vi "Parse-end-tag-2.vi"(6 "State data in":T1, 8 "error in (no error)":errorcluster, 10 "String in":string, 11 "Element-XML in":refnum<class "Element-XML.lvclass">) -> (0 "error out":errorcluster, 1 "Valid element?":bool, 2 "Remaining string":string, 3 "Element-XML":refnum<class "Element-XML.lvclass">, 4 "State data":T1)   [LabVIEW 2013, in "HardwareCharacterization.lvlib" / "Element-XML.lvclass"]
uses:
  Element-XML.lvclass
  XML-parser-state.ctl
  Element-XML.lvclass/Element-XML.ctl
  Read Parent ItemID.vi
  Read Element.vi
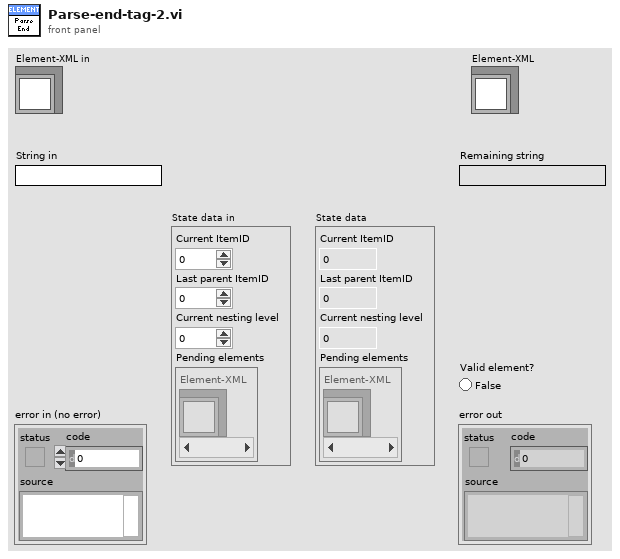
[diagram p1: front panel]
types:
  T1 = typedef "HardwareCharacterization.lvlib/Element-XML.lvclass/XML-parser-state.ctl" = cluster{"Current ItemID":u32, "Last parent ItemID":u32, "Current nesting level":i16, "Pending elements":refnum<class "Element-XML.lvclass">[]}
  T2 = typedef "HardwareCharacterization.lvlib/Element-XML.lvclass/Elements.ctl" = enum16{"BeginJob", "WriteDigital", "WriteAnalog", "Set", "ApplicationEvent", "JumpAbs", "MarkAbs", "JumpRel", "MarkRel", "LongDelay", "EndJob"}
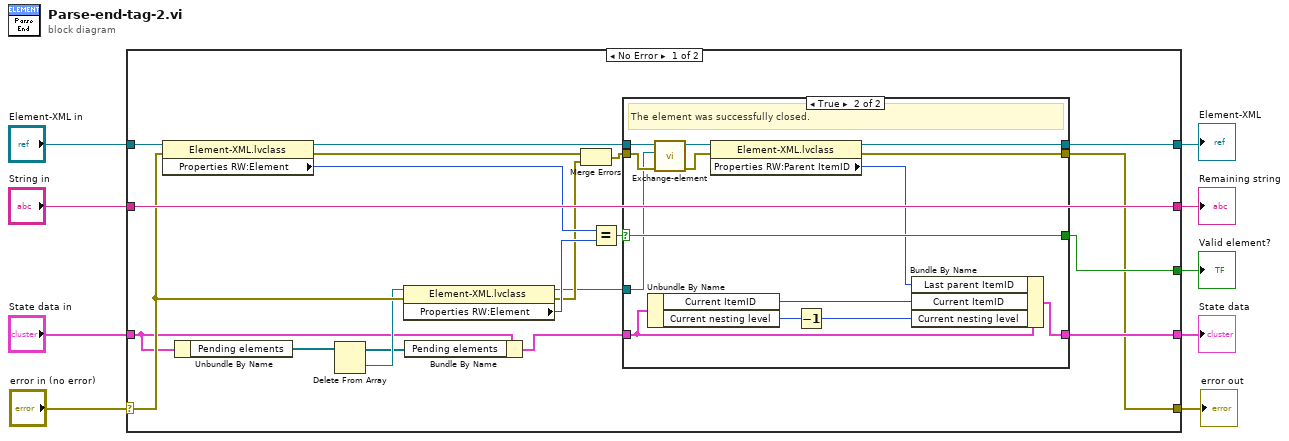
[diagram p0: block diagram]
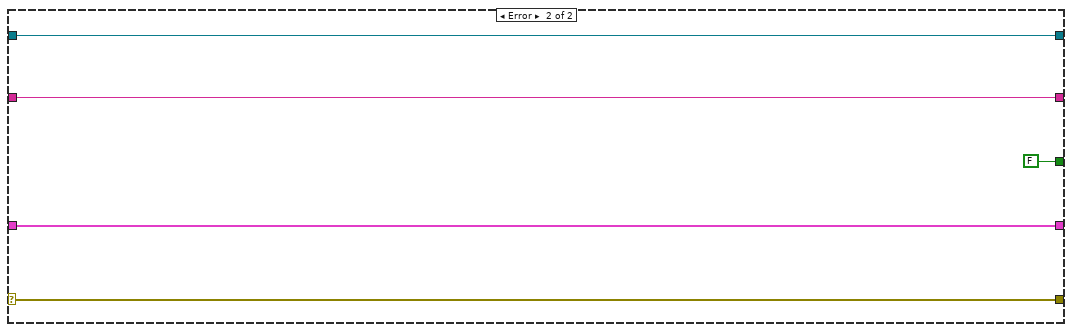
[diagram p3: hidden frame]
diagram:
  n1 = case shown="No Error" "error in (no error)" {
    selector: "error in (no error)" -> [w16 w52]
    tunnel: [w15 w52] -> w8
    tunnel: [w24 w51] -> w2
    tunnel: "Element-XML in" -> [w27 w51]
    tunnel: "String in" -> [w29 w50]
    tunnel: [w29 w50] -> w6
    tunnel: "State data in" -> [w11 w49]
    tunnel: [w22 w49] -> w4
    tunnel: [w17 FALSE] -> w1
    frame No Error {
      n2 = property class="Element-XML.lvclass"(reference=w27, error in=w16) -> (reference out=w25:refnum<class "Element-XML.lvclass">, error out=w20:errorcluster, "Properties RW:Element"=w28:T2)
      n3 = Unbundle By Name(w11) -> ("Pending elements"=w14:refnum<class "Element-XML.lvclass">[])
      n4 = Delete From Array(array=w14) -> (deleted portion=w13:refnum<class "Element-XML.lvclass">, array with subset deleted=w12:refnum<class "Element-XML.lvclass">[])  [unwired: 2 in]
      n5 = property class="Element-XML.lvclass"(reference=w13, error in=w16) -> (reference out=w18:refnum<class "Element-XML.lvclass">, error out=w19:errorcluster, "Properties RW:Element"=w26:T2)
      n6 = Bundle By Name(cluster=w11, "Pending elements"=w12) -> (w10:T1)
      n7 = Merge Errors(w20, w19) -> (w21:errorcluster)
      n8 = Equal?(x=w28, y=w26) -> (x = y?=w23:bool)
      n9 = case shown="True" w23 {
        selector: w23 -> [w31 w44]
        tunnel: w10 -> [w30 w43]
        tunnel: [w30 w47] -> w22
        tunnel: w25 -> [w33 w42]
        tunnel: w21 -> [w32 w40]
        tunnel: [w33 w46] -> w24
        tunnel: [w32 w45] -> w15
        tunnel: [w31 w44] -> w17
        tunnel: w18 -> [_ w39]
        frame False {
          # "No matching closing tag = syntax error."
        }
        frame True {
          # "The element was successfully closed."
          n10 = Unbundle By Name(w43) -> ("Current ItemID"=w34:u32, "Current nesting level"=w37:i16)
          n11 = call "Exchange-element.vi"("error in (no error)"=w40, "Element-XML in 2"=w39, "Element-XML in"=w42) -> ("error out"=w38:errorcluster, "Element-XML out"=w41:refnum<class "Element-XML.lvclass">)  [unwired: 6 in, 1 out]
          n12 = property class="Element-XML.lvclass"(reference=w41, error in=w38) -> (reference out=w46:refnum<class "Element-XML.lvclass">, error out=w45:errorcluster, "Properties RW:Parent ItemID"=w35:u32)
          n13 = Decrement(x=w37) -> (x-1=w36:i16)
          n14 = Bundle By Name(cluster=w43, "Last parent ItemID"=w35, "Current ItemID"=w34, "Current nesting level"=w36) -> (w47:T1)
        }
      }
    }
    frame Error {
    }
  }
  "error out" <- w8
  "State data" <- w4
  "Valid element?" <- w1
  "Remaining string" <- w6
  "Element-XML" <- w2
